vi "Helper commandTimeout.vi"(8 "error in (no error)":errorcluster, 11 "commandTimeout in":i32=-1) -> (0 "error out":errorcluster, 3 ".NET Refnum out":refnum<k24>)   [LabVIEW 2020, in "ORM_Dapper.lvlib" / "DapperMapper.lvclass"]
uses:
  DapperMapper.lvclass
  DapperMapper.lvclass/DapperMapper.ctl
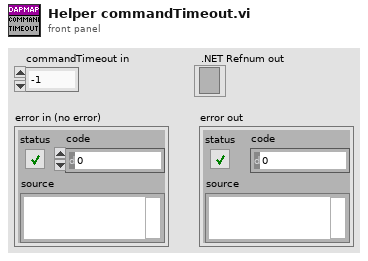
[diagram p1: front panel]
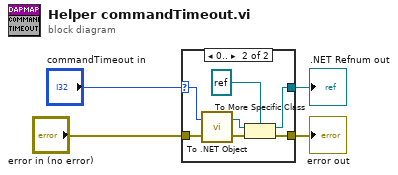
[diagram p0: block diagram]
diagram:
  n1 = case shown="0.." "commandTimeout in" {
    selector: "commandTimeout in" -> [_ w12]
    tunnel: [_ w10] -> w2
    tunnel: "error in (no error)" -> [w5 w7]
    tunnel: [w5 w6] -> w4
    frame Default {
    }
    frame 0.. {
      n2 = call <vilib>:"To .NET Object.vi"("error in (no error)"=w7, "anything"=w12) -> ("error out"=w8:errorcluster, ".NET object"=w9:refnum<k24>)
      n3 = To More Specific Class(target class=refnum<k24> refnum ("commandTimeout"), reference=w9, error in=w8) -> (specific class reference=w10:refnum<k24>, error out=w6:errorcluster)
    }
  }
  "error out" <- w4
  ".NET Refnum out" <- w2
